vi "Monitoring task.vi"   [LabVIEW 2016, in "PLC.lvlib"]
uses:
  PLC.lvlib
types:
  T1 = cluster{"测试模式":enum16{"正常测试", "集成干预"}, "参数启用":cluster{"氨氮":bool, "总磷":bool, "总氮":bool, "多参数":bool, "CODMn":bool, "CODcr":bool, "超标留样":bool}}
  T2 = enum16{"加标流程（润洗/采样分开）", "加标流程（润洗/采样合并）", "加标流程（不启动采配水）", "水样测试（润洗/采样分开）", "水样测试（润洗/采样合并）", "水样测试（不启动采配水）"}
  T3 = cluster{"氨氮":bool, "总磷":bool, "总氮":bool, "多参数":bool, "CODMn":bool, "CODcr":bool, "超标留样":bool}
  T4 = typedef "质控单元V4.lvlib/质控slave id.ctl" = enum16{"null", "氨氮", "总磷", "总氮", "CODMn", "CODCr", "氨氮总磷", "总磷总氮"}
  T5 = cluster{"时间标识":timestamp, "参数":string, "数据类型":string, "集成干预测试浓度值":dbl, "集成干预前测试时间":timestamp, "集成干预前测试浓度值":dbl}
  T6 = enum32{"Bad", "Idle", "Run top level", "Running"}
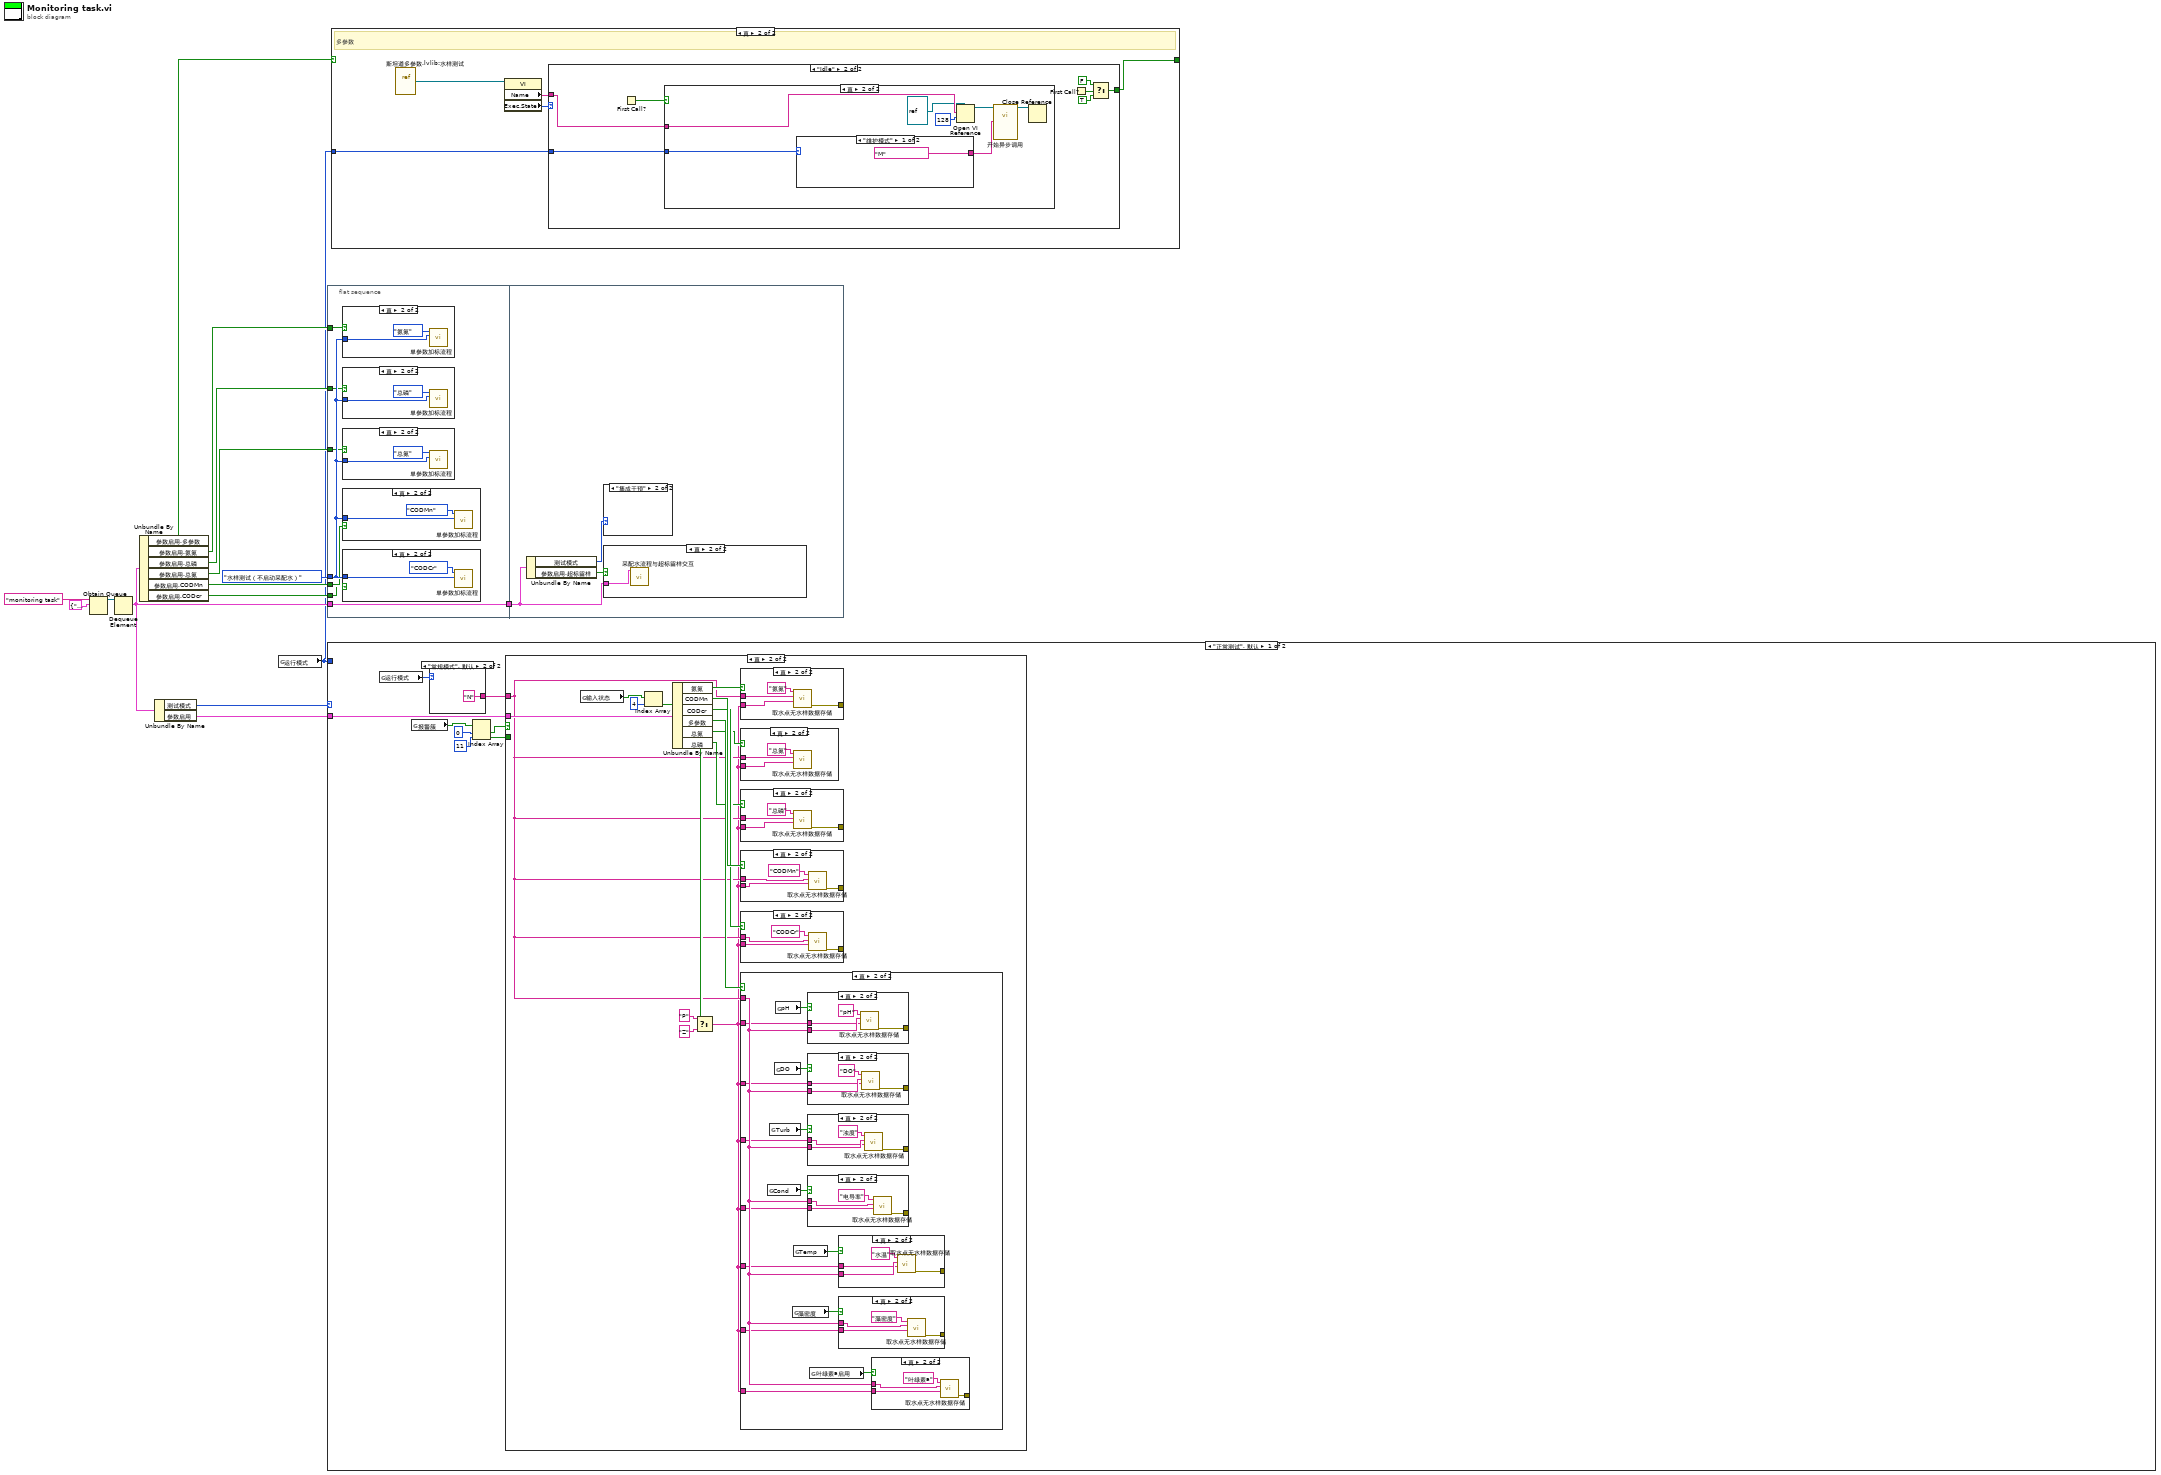
[diagram p0: block diagram]
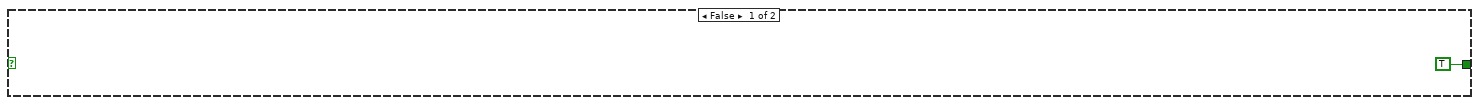
[diagram p2: hidden frame]
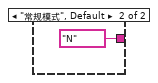
[diagram p5: hidden frame]
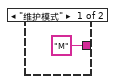
[diagram p6: hidden frame]
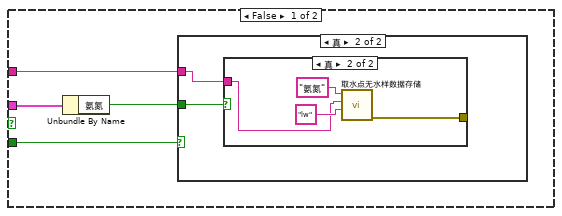
[diagram p7: hidden frame]
diagram:
  n1 = Obtain Queue(name (unnamed)="monitoring task" ("名称（未命名）"), element data type=T1 {"测试模式"=enum."正常测试", "参数启用"={"氨氮"=FALSE, "总磷"=FALSE, "总氮"=FALSE, "多参数"=FALSE, "CODMn"=FALSE, "CODcr"=FALSE, "超标留样"=FALSE}} ("参数")) -> (queue out=w12:refnum<queue>)  [unwired: 3 in, 2 out]
  n2 = Dequeue Element(queue=w12) -> (element=w5:T1)  [unwired: 2 in, 3 out]
  n3 = Unbundle By Name(w5) -> ("参数启用.多参数"=w2:bool, "参数启用.氨氮"=w11:bool, "参数启用.总磷"=w10:bool, "参数启用.总氮"=w9:bool, "参数启用.CODMn"=w8:bool, "参数启用.CODcr"=w7:bool)
  n4 = Unbundle By Name(w5) -> ("测试模式"=w3:enum16{"正常测试", "集成干预"}, "参数启用"=w4:T3)
  n5 = global read "系统设置全局变量.vi" "运行模式"() -> (w1:enum16{"维护模式", "常规模式", "应急模式", "质控模式"})
  n6 = flat-sequence {
    tunnel: T2."水样测试（不启动采配水）" ("流程类型") -> [w22]
    tunnel: w11 -> [w21]
    tunnel: w10 -> [w20]
    tunnel: w9 -> [w19]
    tunnel: w8 -> [w18]
    tunnel: w7 -> [w17]
    tunnel: [w16] -> w6
    tunnel: w5 -> [w16]
    tunnel: w6 -> [w35]
    frame #0 {
      n7 = case shown="真" w21 {
        tunnel: w22 -> [_ w31]
        frame False {
        }
        frame True {
          n8 = call "单参数加标流程.vi"("流程类型"=w31, "Slave ID"=质控slave_id."氨氮") -> ()  [unwired: 10 in]
        }
      }
      n9 = case shown="真" w20 {
        tunnel: w22 -> [_ w29]
        frame False {
        }
        frame True {
          n10 = call "单参数加标流程.vi"("流程类型"=w29, "Slave ID"=质控slave_id."总磷") -> ()  [unwired: 10 in]
        }
      }
      n11 = case shown="真" w19 {
        tunnel: w22 -> [_ w27]
        frame False {
        }
        frame True {
          n12 = call "单参数加标流程.vi"("流程类型"=w27, "Slave ID"=质控slave_id."总氮") -> ()  [unwired: 10 in]
        }
      }
      n13 = case shown="真" w18 {
        tunnel: w22 -> [_ w25]
        frame False {
        }
        frame True {
          n14 = call "单参数加标流程.vi"("流程类型"=w25, "Slave ID"=质控slave_id."CODMn") -> ()  [unwired: 10 in]
        }
      }
      n15 = case shown="真" w17 {
        tunnel: w22 -> [_ w23]
        frame False {
        }
        frame True {
          n16 = call "单参数加标流程.vi"("流程类型"=w23, "Slave ID"=质控slave_id."CODCr") -> ()  [unwired: 10 in]
        }
      }
    }
    frame #1 {
      n17 = Unbundle By Name(w35) -> ("测试模式"=w33:enum16{"正常测试", "集成干预"}, "参数启用.超标留样"=w34:bool)
      n18 = case shown="\"集成干预\"" w33 {
        frame "正常测试", Default {
        }
        frame "集成干预" {
        }
      }
      n19 = case shown="真" w34 {
        tunnel: w35 -> [_ w36]
        frame False {
        }
        frame True {
          n20 = call "采配水流程与超标留样交互.vi"("参数"=w36) -> ()  [unwired: 11 in]
        }
      }
    }
  }
  n21 = case shown="\"正常测试\", 默认" w3 {
    tunnel: w4 -> [w39 w145]
    tunnel: w1 -> [_ w133]
    frame "正常测试", Default {
      n22 = global read "系统设置全局变量.vi" "运行模式"() -> (w37:enum16{"维护模式", "常规模式", "应急模式", "质控模式"})
      n23 = global read "采配水全局变量.vi" "报警簇"() -> (w44:bool[])
      n24 = case shown="\"常规模式\", 默认" w37 {
        tunnel: ["M" ("table") "N" ("table")] -> w38
        frame "维护模式" {
        }
        frame "常规模式", Default {
        }
      }
      n25 = Index Array(array=w44, index #1=0 ("索引"), index #2=11 ("索引")) -> (element #1=w41:bool, element #2=w40:bool)
      n26 = case shown="真" w41 {
        tunnel: w40 -> [w50 _]
        tunnel: w39 -> [w49 w70]
        tunnel: w38 -> [w47 w58]
        frame False {
          n27 = Unbundle By Name(w49) -> ("氨氮"=w48:bool)
          n28 = case shown="真" w50 {
            tunnel: w48 -> [_ w52]
            tunnel: w47 -> [_ w51]
            frame False {
            }
            frame True {
              n29 = case shown="真" w52 {
                tunnel: w51 -> [_ w53]
                tunnel: [_ w54] -> _
                frame False {
                }
                frame True {
                  n30 = call "取水点无水样数据存储.vi"("数据标识"="lw", "数据类型"=w53, "table"="氨氮") -> ("error out"=w54:errorcluster)  [unwired: 8 in]
                }
              }
            }
          }
        }
        frame True {
          n31 = global read "采配水全局变量.vi" "输入状态"() -> (w63:bool[])
          n32 = Index Array(array=w63, index=4 ("索引")) -> (element=w61:bool)
          n33 = Unbundle By Name(w70) -> ("氨氮"=w69:bool, "CODMn"=w68:bool, "CODcr"=w67:bool, "多参数"=w66:bool, "总氮"=w65:bool, "总磷"=w64:bool)
          n34 = Select(t="P" ("数据标识"), s=w61, f="Z" ("数据标识")) -> (s? t:f=w57:string)
          n35 = case shown="真" w69 {
            tunnel: w58 -> [_ w130]
            tunnel: [_ w131] -> _
            tunnel: w57 -> [_ w129]
            frame False {
            }
            frame True {
              n36 = call "取水点无水样数据存储.vi"("数据标识"=w129, "数据类型"=w130, "table"="氨氮") -> ("error out"=w131:errorcluster)  [unwired: 8 in]
            }
          }
          n37 = case shown="真" w65 {
            tunnel: w58 -> [_ w76]
            tunnel: w57 -> [_ w75]
            frame False {
            }
            frame True {
              n38 = call "取水点无水样数据存储.vi"("数据标识"=w75, "数据类型"=w76, "table"="总氮") -> ()  [unwired: 8 in, 1 out]
            }
          }
          n39 = case shown="真" w64 {
            tunnel: [_ w73] -> _
            tunnel: w57 -> [_ w72]
            tunnel: w58 -> [_ w71]
            frame False {
            }
            frame True {
              n40 = call "取水点无水样数据存储.vi"("数据标识"=w72, "数据类型"=w71, "table"="总磷") -> ("error out"=w73:errorcluster)  [unwired: 8 in]
            }
          }
          n41 = case shown="真" w68 {
            tunnel: w58 -> [_ w127]
            tunnel: [_ w126] -> _
            tunnel: w57 -> [_ w125]
            frame False {
            }
            frame True {
              n42 = call "取水点无水样数据存储.vi"("数据标识"=w125, "数据类型"=w127, "table"="CODMn") -> ("error out"=w126:errorcluster)  [unwired: 8 in]
            }
          }
          n43 = case shown="真" w67 {
            tunnel: w58 -> [_ w123]
            tunnel: [_ w122] -> _
            tunnel: w57 -> [_ w121]
            frame False {
            }
            frame True {
              n44 = call "取水点无水样数据存储.vi"("数据标识"=w121, "数据类型"=w123, "table"="CODCr") -> ("error out"=w122:errorcluster)  [unwired: 8 in]
            }
          }
          n45 = case shown="真" w66 {
            tunnel: w58 -> [_ w92]
            tunnel: w57 -> [_ w84]
            tunnel: w57 -> [_ w83]
            tunnel: w57 -> [_ w82]
            tunnel: w57 -> [_ w81]
            tunnel: w57 -> [_ w80]
            tunnel: w57 -> [_ w79]
            tunnel: w57 -> [_ w78]
            frame False {
            }
            frame True {
              n46 = global read "断电保存变量.vi" "Cond"() -> (w87:bool)
              n47 = global read "断电保存变量.vi" "Turb"() -> (w88:bool)
              n48 = global read "断电保存变量.vi" "DO"() -> (w89:bool)
              n49 = global read "断电保存变量.vi" "pH"() -> (w90:bool)
              n50 = global read "断电保存变量.vi" "藻密度"() -> (w85:bool)
              n51 = global read "断电保存变量.vi" "Temp"() -> (w91:bool)
              n52 = case shown="真" w90 {
                tunnel: w92 -> [_ w115]
                tunnel: [_ w114] -> _
                tunnel: w84 -> [_ w113]
                frame False {
                }
                frame True {
                  n53 = call "取水点无水样数据存储.vi"("数据标识"=w113, "数据类型"=w115, "table"="pH") -> ("error out"=w114:errorcluster)  [unwired: 8 in]
                }
              }
              n54 = case shown="真" w89 {
                tunnel: w92 -> [_ w111]
                tunnel: [_ w110] -> _
                tunnel: w83 -> [_ w109]
                frame False {
                }
                frame True {
                  n55 = call "取水点无水样数据存储.vi"("数据标识"=w109, "数据类型"=w111, "table"="DO") -> ("error out"=w110:errorcluster)  [unwired: 8 in]
                }
              }
              n56 = case shown="真" w88 {
                tunnel: w92 -> [_ w103]
                tunnel: [_ w102] -> _
                tunnel: w82 -> [_ w101]
                frame False {
                }
                frame True {
                  n57 = call "取水点无水样数据存储.vi"("数据标识"=w101, "数据类型"=w103, "table"="浊度") -> ("error out"=w102:errorcluster)  [unwired: 8 in]
                }
              }
              n58 = case shown="真" w87 {
                tunnel: w92 -> [_ w107]
                tunnel: [_ w106] -> _
                tunnel: w80 -> [_ w105]
                frame False {
                }
                frame True {
                  n59 = call "取水点无水样数据存储.vi"("数据标识"=w105, "数据类型"=w107, "table"="电导率") -> ("error out"=w106:errorcluster)  [unwired: 8 in]
                }
              }
              n60 = global read "断电保存变量.vi" "叶绿素a启用"() -> (w86:bool)
              n61 = case shown="真" w91 {
                tunnel: w92 -> [_ w119]
                tunnel: [_ w118] -> _
                tunnel: w81 -> [_ w117]
                frame False {
                }
                frame True {
                  n62 = call "取水点无水样数据存储.vi"("数据标识"=w117, "数据类型"=w119, "table"="水温") -> ("error out"=w118:errorcluster)  [unwired: 8 in]
                }
              }
              n63 = case shown="真" w85 {
                tunnel: w92 -> [_ w95]
                tunnel: [_ w94] -> _
                tunnel: w79 -> [_ w93]
                frame False {
                }
                frame True {
                  n64 = call "取水点无水样数据存储.vi"("数据标识"=w93, "数据类型"=w95, "table"="藻密度") -> ("error out"=w94:errorcluster)  [unwired: 8 in]
                }
              }
              n65 = case shown="真" w86 {
                tunnel: w92 -> [_ w99]
                tunnel: [_ w98] -> _
                tunnel: w78 -> [_ w97]
                frame False {
                }
                frame True {
                  n66 = call "取水点无水样数据存储.vi"("数据标识"=w97, "数据类型"=w99, "table"="叶绿素a") -> ("error out"=w98:errorcluster)  [unwired: 8 in]
                }
              }
            }
          }
        }
      }
    }
    frame "集成干预" {
      n67 = Unbundle By Name(w145) -> ("总磷"=w139:bool, "总氮"=w140:bool, "氨氮"=w144:bool, "CODMn"=w143:bool, "CODcr"=w142:bool, "多参数"=w141:bool)
      n68 = case shown="真" w139 {
        tunnel: [_ w152] -> w138
        tunnel: w133 -> [_ w151]
        frame False {
        }
        frame True {
          n69 = call "获取最近两组水样测试数据.vi"("运行模式"=w151, "table"="总磷") -> ("error out"=w155:errorcluster, "存储变量"=w154:T5)  [unwired: 8 in]
          n70 = call "集成干预测试数据存储.vi"("error in (no error)"=w155, "存储变量"=w154) -> ("error out"=w152:errorcluster)  [unwired: 9 in]
        }
      }
      n71 = case shown="真" w140 {
        tunnel: w138 -> [_ _]
        tunnel: [_ w147] -> w137
        tunnel: w133 -> [_ w146]
        frame False {
        }
        frame True {
          n72 = call "获取最近两组水样测试数据.vi"("运行模式"=w146, "table"="总氮") -> ("error out"=w150:errorcluster, "存储变量"=w149:T5)  [unwired: 8 in]
          n73 = call "集成干预测试数据存储.vi"("error in (no error)"=w150, "存储变量"=w149) -> ("error out"=w147:errorcluster)  [unwired: 9 in]
        }
      }
      n74 = case shown="真" w144 {
        tunnel: w137 -> [_ _]
        tunnel: [_ w216] -> w134
        tunnel: w133 -> [_ w215]
        frame False {
        }
        frame True {
          n75 = call "获取最近两组水样测试数据.vi"("运行模式"=w215, "table"="氨氮") -> ("error out"=w217:errorcluster, "存储变量"=w218:T5)  [unwired: 8 in]
          n76 = call "集成干预测试数据存储.vi"("error in (no error)"=w217, "存储变量"=w218) -> ("error out"=w216:errorcluster)  [unwired: 9 in]
        }
      }
      n77 = case shown="真" w143 {
        tunnel: [_ w211] -> w136
        tunnel: w134 -> [_ _]
        tunnel: w133 -> [_ w210]
        frame False {
        }
        frame True {
          n78 = call "获取最近两组水样测试数据.vi"("运行模式"=w210, "table"="CODMn") -> ("error out"=w212:errorcluster, "存储变量"=w213:T5)  [unwired: 8 in]
          n79 = call "集成干预测试数据存储.vi"("error in (no error)"=w212, "存储变量"=w213) -> ("error out"=w211:errorcluster)  [unwired: 9 in]
        }
      }
      n80 = case shown="真" w142 {
        tunnel: w136 -> [_ _]
        tunnel: [_ w206] -> w135
        frame False {
        }
        frame True {
          n81 = global read "系统设置全局变量.vi" "运行模式"() -> (w205:enum16{"维护模式", "常规模式", "应急模式", "质控模式"})
          n82 = call "获取最近两组水样测试数据.vi"("运行模式"=w205, "table"="CODCr") -> ("error out"=w207:errorcluster, "存储变量"=w208:T5)  [unwired: 8 in]
          n83 = call "集成干预测试数据存储.vi"("error in (no error)"=w207, "存储变量"=w208) -> ("error out"=w206:errorcluster)  [unwired: 9 in]
        }
      }
      n84 = case shown="真" w141 {
        tunnel: w135 -> [_ _]
        tunnel: w133 -> [_ w156]
        frame False {
        }
        frame True {
          n85 = global read "断电保存变量.vi" "Temp"() -> (w163:bool)
          n86 = case shown="真" w163 {
            tunnel: [_ w201] -> w169
            tunnel: w156 -> [_ w200]
            frame False {
            }
            frame True {
              n87 = call "获取最近两组水样测试数据.vi"("运行模式"=w200, "table"="水温") -> ("error out"=w204:errorcluster, "存储变量"=w203:T5)  [unwired: 8 in]
              n88 = call "集成干预测试数据存储.vi"("error in (no error)"=w204, "存储变量"=w203) -> ("error out"=w201:errorcluster)  [unwired: 9 in]
            }
          }
          n89 = global read "断电保存变量.vi" "pH"() -> (w162:bool)
          n90 = case shown="真" w162 {
            tunnel: [_ w196] -> w168
            tunnel: w169 -> [_ _]
            tunnel: w156 -> [_ w195]
            frame False {
            }
            frame True {
              n91 = call "获取最近两组水样测试数据.vi"("运行模式"=w195, "table"="pH") -> ("error out"=w199:errorcluster, "存储变量"=w198:T5)  [unwired: 8 in]
              n92 = call "集成干预测试数据存储.vi"("error in (no error)"=w199, "存储变量"=w198) -> ("error out"=w196:errorcluster)  [unwired: 9 in]
            }
          }
          n93 = global read "断电保存变量.vi" "DO"() -> (w161:bool)
          n94 = case shown="真" w161 {
            tunnel: [_ w191] -> w167
            tunnel: w168 -> [_ _]
            tunnel: w156 -> [_ w190]
            frame False {
            }
            frame True {
              n95 = call "获取最近两组水样测试数据.vi"("运行模式"=w190, "table"="DO") -> ("error out"=w194:errorcluster, "存储变量"=w193:T5)  [unwired: 8 in]
              n96 = call "集成干预测试数据存储.vi"("error in (no error)"=w194, "存储变量"=w193) -> ("error out"=w191:errorcluster)  [unwired: 9 in]
            }
          }
          n97 = global read "断电保存变量.vi" "Cond"() -> (w160:bool)
          n98 = case shown="真" w160 {
            tunnel: [_ w186] -> w166
            tunnel: w167 -> [_ _]
            tunnel: w156 -> [_ w185]
            frame False {
            }
            frame True {
              n99 = call "获取最近两组水样测试数据.vi"("运行模式"=w185, "table"="电导率") -> ("error out"=w189:errorcluster, "存储变量"=w188:T5)  [unwired: 8 in]
              n100 = call "集成干预测试数据存储.vi"("error in (no error)"=w189, "存储变量"=w188) -> ("error out"=w186:errorcluster)  [unwired: 9 in]
            }
          }
          n101 = global read "断电保存变量.vi" "Turb"() -> (w159:bool)
          n102 = case shown="真" w159 {
            tunnel: [_ w181] -> w165
            tunnel: w166 -> [_ _]
            tunnel: w156 -> [_ w180]
            frame False {
            }
            frame True {
              n103 = call "获取最近两组水样测试数据.vi"("运行模式"=w180, "table"="浊度") -> ("error out"=w184:errorcluster, "存储变量"=w183:T5)  [unwired: 8 in]
              n104 = call "集成干预测试数据存储.vi"("error in (no error)"=w184, "存储变量"=w183) -> ("error out"=w181:errorcluster)  [unwired: 9 in]
            }
          }
          n105 = global read "断电保存变量.vi" "叶绿素a启用"() -> (w158:bool)
          n106 = case shown="真" w158 {
            tunnel: [_ w176] -> w164
            tunnel: w165 -> [_ _]
            tunnel: w156 -> [_ w175]
            frame False {
            }
            frame True {
              n107 = call "获取最近两组水样测试数据.vi"("运行模式"=w175, "table"="叶绿素a") -> ("error out"=w179:errorcluster, "存储变量"=w178:T5)  [unwired: 8 in]
              n108 = call "集成干预测试数据存储.vi"("error in (no error)"=w179, "存储变量"=w178) -> ("error out"=w176:errorcluster)  [unwired: 9 in]
            }
          }
          n109 = global read "断电保存变量.vi" "藻密度"() -> (w157:bool)
          n110 = case shown="真" w157 {
            tunnel: [_ w171] -> _
            tunnel: w164 -> [_ _]
            tunnel: w156 -> [_ w170]
            frame False {
            }
            frame True {
              n111 = call "获取最近两组水样测试数据.vi"("运行模式"=w170, "table"="藻密度") -> ("error out"=w174:errorcluster, "存储变量"=w173:T5)  [unwired: 8 in]
              n112 = call "集成干预测试数据存储.vi"("error in (no error)"=w174, "存储变量"=w173) -> ("error out"=w171:errorcluster)  [unwired: 9 in]
            }
          }
        }
      }
    }
  }
  n113 = case shown="真" w2 {
    tunnel: [TRUE ("t") w225] -> _
    tunnel: w1 -> [_ w221]
    frame False {
    }
    frame True {
      # "多参数"
      n114 = vi-ref "斯坦道多参数.lvlib:水样测试.vi"() -> (w223:refnum<vi>)
      n115 = property class="VI"(reference=w223) -> ("Name"=w222:string, "Exec.State"=w224:T6)  [unwired: 1 in, 2 out]
      n116 = case shown="\"Idle\"" w224 {
        tunnel: w222 -> [_ w232]
        tunnel: [_ w227] -> w225
        tunnel: w221 -> [_ w226]
        frame "Bad", Default {
        }
        frame "Idle" {
          n117 = First Call?() -> (First Call?: T/F=w231:bool)
          n118 = case shown="真" w231 {
            tunnel: w232 -> [_ w238]
            tunnel: w226 -> [_ w233]
            frame False {
            }
            frame True {
              n119 = case shown="\"维护模式\"" w233 {
                tunnel: ["M" ("数据标记表") "N" ("数据标记表")] -> w235
                frame "维护模式" {
                }
                frame "常规模式", Default {
                }
              }
              n120 = Open VI Reference(type specifier VI Refnum (for type only)=refnum<vi> refnum, vi path=w238, options=128 ("选项")) -> (vi reference=w237:refnum<vi>)  [unwired: 3 in, 1 out]
              n121 = call-by-ref "开始异步调用"(reference=w237, "数据标记表"=w235) -> (reference out=w236:refnum<vi>)  [unwired: 12 in, 1 out]
              n122 = Close Reference(reference=w236) -> ()  [unwired: 1 in, 1 out]
            }
          }
          n123 = First Call?() -> (First Call?: T/F=w230:bool)
          n124 = Select(t=FALSE, s=w230, f=TRUE) -> (s? t:f=w227:bool)
        }
      }
    }
  }
